vi "ANNUNCIATOR.vi"(5 "Input Channel":T1(ring), 6 "Input Value":bool) -> (0 "Out Warning OverPressure":bool, 1 "Out Warning OverTemp":bool, 2 "Out Caution 3":bool, 3 "Out Caution 2":bool, 4 "Out Caution Data":bool)   [LabVIEW 2013]
doc: "Allows for setting or reading the annunciator values from anywhere in the calling VI. More of a simple singleton than a proper action engine."
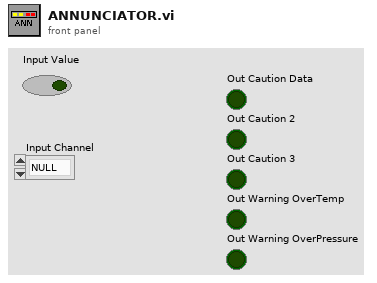
[diagram p1: front panel]
types:
  T1 = enum16{"NULL", "Caution Data", "Caution 2", "Caution 3", "Warning OverTemp", "Warning OverPressure"}
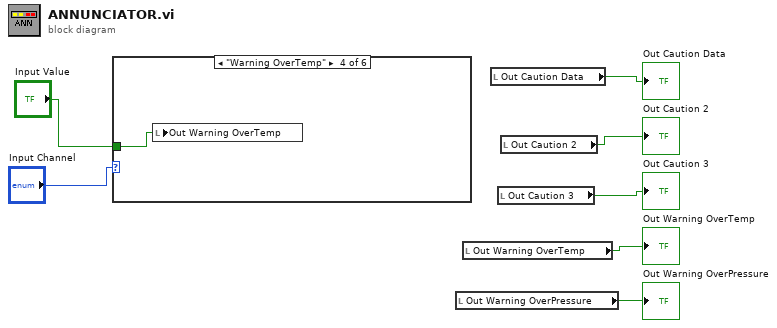
[diagram p0: block diagram]
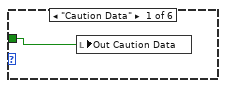
[diagram p2: hidden frame]
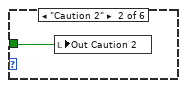
[diagram p3: hidden frame]
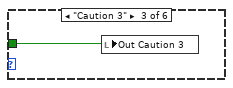
[diagram p4: hidden frame]
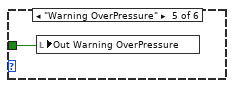
[diagram p5: hidden frame]
diagram:
  n1 = case shown="\"Warning OverTemp\"" "Input Channel" {
    tunnel: "Input Value" -> [w8 w9 w10 w11 w12 _]
    frame "Caution Data" {
      n2 = local write "Out Caution Data"(w8) -> ()
    }
    frame "Caution 2" {
      n3 = local write "Out Caution 2"(w9) -> ()
    }
    frame "Caution 3" {
      n4 = local write "Out Caution 3"(w10) -> ()
    }
    frame "Warning OverTemp" {
      n5 = local write "Out Warning OverTemp"(w11) -> ()
    }
    frame "Warning OverPressure" {
      n6 = local write "Out Warning OverPressure"(w12) -> ()
    }
    frame "NULL", Default {
    }
  }
  n7 = local read "Out Warning OverPressure"() -> (→"Out Warning OverPressure":bool)
  n8 = local read "Out Warning OverTemp"() -> (→"Out Warning OverTemp":bool)
  n9 = local read "Out Caution Data"() -> (→"Out Caution Data":bool)
  n10 = local read "Out Caution 3"() -> (→"Out Caution 3":bool)
  n11 = local read "Out Caution 2"() -> (→"Out Caution 2":bool)
